vi "New Input Poller Queue.vi"(8 "error in (no error)":errorcluster) -> (0 "error out":errorcluster, 2 "listen_result_queue":refnum<queue>, 3 "input poller":refnum<class "input_poller_queue.lvclass">)   [LabVIEW 2015, in "input_poller_queue.lvclass"]
uses:
  input_poller_queue.lvclass
  Result/result.lvclass
  input_poller_queue.lvclass/input_poller_queue.ctl
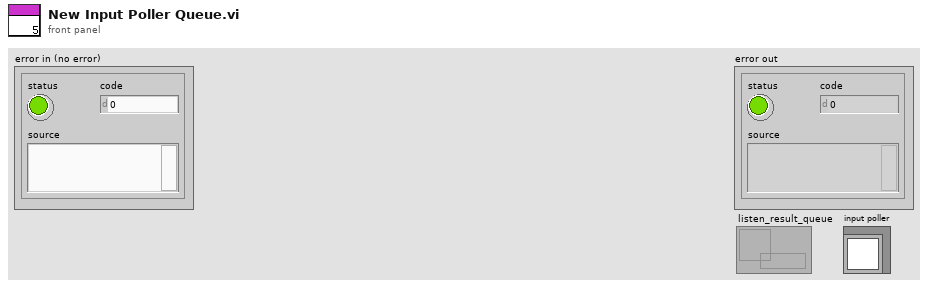
[diagram p1: front panel]
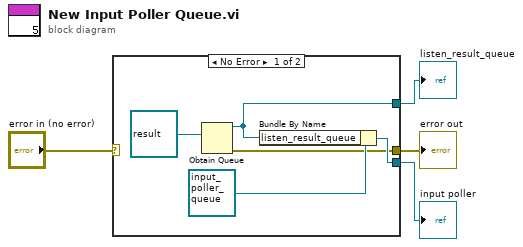
[diagram p0: block diagram]
diagram:
  n1 = case shown="No Error" "error in (no error)" {
    selector: "error in (no error)" -> [_ w10]
    tunnel: [w7 _] -> w3
    tunnel: [w6 _] -> w2
    tunnel: [w5 w10] -> w1
    frame No Error {
      n2 = Obtain Queue(element data type=refnum<class "result.lvclass"> refnum ("result.lvclass")) -> (queue out=w7:refnum<queue>, error out=w5:errorcluster)  [unwired: 4 in, 1 out]
      n3 = Bundle By Name(cluster=refnum<class "input_poller_queue.lvclass"> refnum ("input_poller_queue.lvclass"), "listen_result_queue"=w7) -> (w6:refnum<class "input_poller_queue.lvclass">)
    }
    frame Error {
    }
  }
  "error out" <- w1
  "listen_result_queue" <- w3
  "input poller" <- w2
